vi "Host_SurfaceMetalGeneration.vi"() -> ()   [LabVIEW 2014]
uses:
  <vilib>/Instr/_visa.llb/VISA Configure Serial Port (Instr).vi
  <vilib>/FPGAPlugInAG/PCIe-7851R/niLvFpga_Open_PCIe-7851R.vi
  <vilib>/rvi/interface/common/dynamic/niFpgaDynamicAddResources.vi
  <vilib>/Utility/error.llb/Error Cluster From Error Code.vi
  <vilib>/rvi/errors/niLvFpgaAdjustHostInterfaceError.vi
  <vilib>/FPGAPlugInAG/Dynamic/niLvFpga_Close_Dynamic.vi
  <vilib>/rvi/interface/nirviOpenFPGA/nirviOpenFPGA.xnode
  FPGA Bitfiles/MetalGrowthv1_FPGATarget_FPGASurfaceSingl_DR9YibpgOIc.lvbitx
  <vilib>/rvi/interface/nirviReadWriteControl/nirviReadWriteControl.xnode
  <vilib>/rvi/interface/nirviMethod/nirviMethod.xnode
  <vilib>/rvi/interface/nirviCloseFPGA/nirviCloseFPGA.xnode
  NiFpgaLv.dll
  <vilib>/rvi/interface/Simulation/niFpgaSimulationCallBeginRW.vi
  <vilib>/FPGAPlugInAG/Dynamic/niLvFpga_ReadFifo_Dynamic.vi
  <vilib>/rvi/errors/niLvFpgaMergeErrorWithErrorCode.vi
panel:
  in  "stop":bool
  in  "DataRequired?":bool
  out "YPos":dbl
  out "XPos":dbl
  in  "XYPIZ":refnum<visa-resource-name>
  in  "GradualWithdraw?":bool
  in  "ZOffset":i32
  in  "StiffLatency":i32
  in  "ThresMultiplier":i32
  in  "OutputVoltIndex":i32
  in  "ZWithdrawStepNum":i32
  in  "ZWithdrawStepIndex":i32
  in  "ZDecStepIndex":i32
  in  "WithdrawLatency us":i32
  in  "MonitorLatency us":i32
  in  "DescendCycle":i32
  in  "YStepNum":i32
  in  "YStepLen um":dbl
  in  "YInitPos um":dbl
  in  "XInitPos um":dbl
  in  "XStepLen um":dbl
  in  "XStepNum":i32
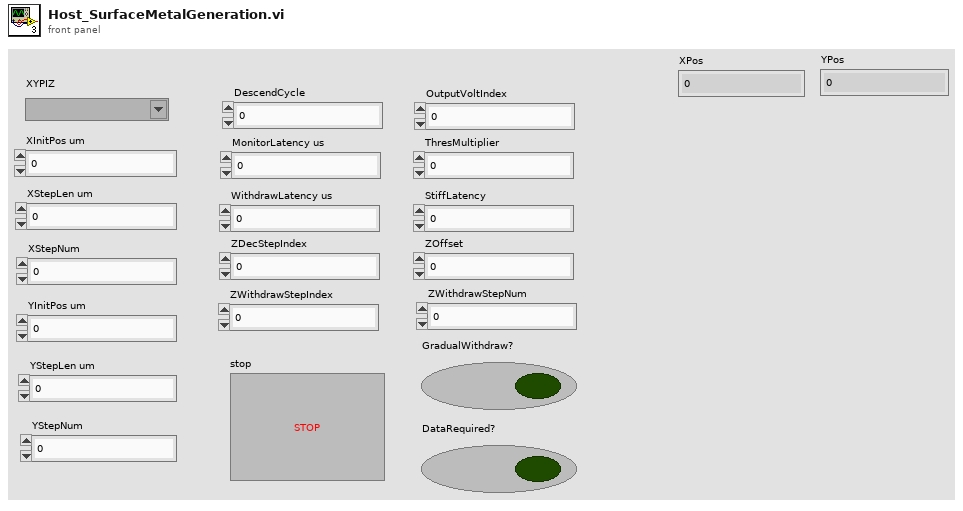
[diagram p1: front panel]
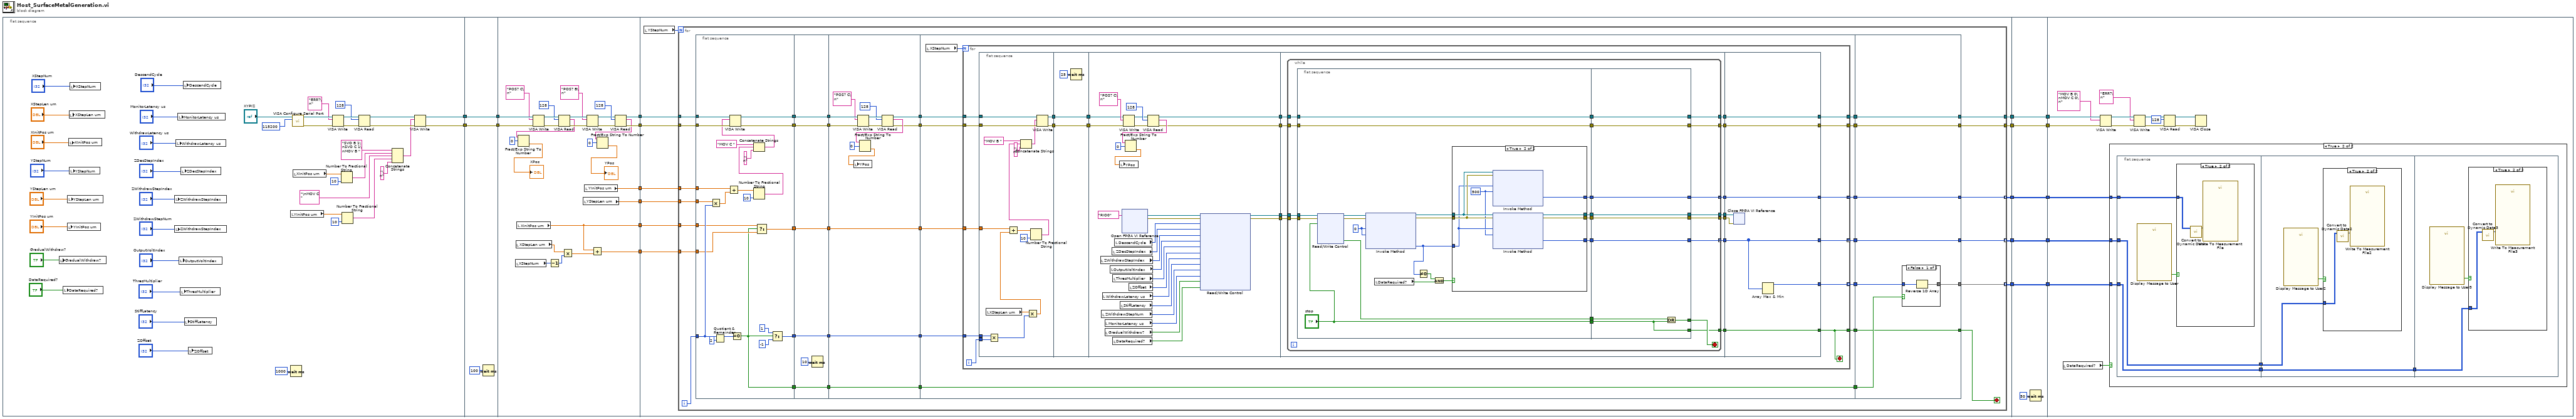
[diagram p0: block diagram]
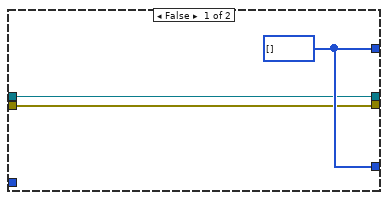
[diagram p2: hidden frame]
diagram:
  n1 = flat-sequence {
    tunnel: [w23] -> w20
    tunnel: [w22] -> w18
    tunnel: w20 -> [w63]
    tunnel: [w63] -> w19
    tunnel: w18 -> [w62]
    tunnel: [w62] -> w17
    tunnel: w19 -> [w92]
    tunnel: w17 -> [w91]
    tunnel: [w80] -> w16
    tunnel: [w79] -> w15
    tunnel: [w65] -> w14
    tunnel: [w69] -> w13
    tunnel: [w68] -> w12
    tunnel: [w67] -> w11
    tunnel: w16 -> [w100]
    tunnel: w15 -> [w99]
    tunnel: w14 -> [w103]
    tunnel: w13 -> [w102]
    tunnel: w12 -> [w101]
    tunnel: w11 -> [w98]
    tunnel: [w97] -> w10
    tunnel: [w96] -> w8
    tunnel: [w95] -> w6
    tunnel: [w94] -> w4
    tunnel: [w93] -> w2
    tunnel: w10 -> [w362]
    tunnel: [w362] -> w9
    tunnel: w8 -> [w361]
    tunnel: [w361] -> w7
    tunnel: w6 -> [w360]
    tunnel: [w360] -> w5
    tunnel: w4 -> [w359]
    tunnel: [w359] -> w3
    tunnel: w2 -> [w358]
    tunnel: [w358] -> w1
    tunnel: w9 -> [w365]
    tunnel: w7 -> [w364]
    tunnel: w5 -> [w363]
    tunnel: w3 -> [w377]
    tunnel: w1 -> [w376]
    frame #0 {
      n2 = local write "GradualWithdraw?"("GradualWithdraw?") -> ()
      n3 = local write "DataRequired?"("DataRequired?") -> ()
      n4 = local write "YInitPos um"("YInitPos um") -> ()
      n5 = local write "YStepLen um"("YStepLen um") -> ()
      n6 = local write "XInitPos um"("XInitPos um") -> ()
      n7 = local write "XStepLen um"("XStepLen um") -> ()
      n8 = local write "YStepNum"("YStepNum") -> ()
      n9 = local write "XStepNum"("XStepNum") -> ()
      n10 = local write "ZWithdrawStepIndex"("ZWithdrawStepIndex") -> ()
      n11 = local write "ZWithdrawStepIndex"("ZWithdrawStepNum") -> ()
      n12 = local write "WithdrawLatency us"("WithdrawLatency us") -> ()
      n13 = local write "MonitorLatency us"("MonitorLatency us") -> ()
      n14 = local write "OutputVoltIndex"("OutputVoltIndex") -> ()
      n15 = local write "ThresMultiplier"("ThresMultiplier") -> ()
      n16 = local write "ZDecStepIndex"("ZDecStepIndex") -> ()
      n17 = local write "DescendCycle"("DescendCycle") -> ()
      n18 = local write "StiffLatency"("StiffLatency") -> ()
      n19 = local write "ZOffset"("ZOffset") -> ()
      n20 = local read "YInitPos um"() -> (w28:dbl)
      n21 = Wait (ms)(milliseconds to wait=u32 1000) -> ()  [unwired: 1 out]
      n22 = call-poly "VISA Configure Serial Port"("VISA resource name"="XYPIZ", "baud rate (9600)"=u32 115200) -> ("VISA resource name out"=w42:refnum<visa-resource-name>, "error out"=w41:errorcluster)  [unwired: 12 in]
      n23 = local read "XInitPos um"() -> (w33:dbl)
      n24 = VISA Write(VISA resource name=w42, write buffer="ERR?\n", error in (no error)=w41) -> (VISA resource name out=w39:refnum<visa-resource-name>, error out=w38:errorcluster)  [unwired: 1 out]
      n25 = Number To Fractional String(number=w33, precision (6)=i16 10) -> (F-format string=w31:string)  [unwired: 2 in]
      n26 = Number To Fractional String(number=w28, precision (6)=i16 10) -> (F-format string=w27:string)  [unwired: 2 in]
      n27 = VISA Read(VISA resource name=w39, byte count=u32 128, error in (no error)=w38) -> (VISA resource name out=w36:refnum<visa-resource-name>, error out=w35:errorcluster)  [unwired: 2 out]
      n28 = Concatenate Strings("SVO B 1\nSVO C 1\nMOV B " ("write buffer"), w31, "\nMOV C " ("string"), w27, "\n" ("string")) -> (w25:string)
      n29 = VISA Write(VISA resource name=w36, write buffer=w25, error in (no error)=w35) -> (VISA resource name out=w23:refnum<visa-resource-name>, error out=w22:errorcluster)  [unwired: 1 out]
    }
    frame #1 {
      n30 = Wait (ms)(milliseconds to wait=u32 100) -> ()  [unwired: 1 out]
    }
    frame #2 {
      n31 = local read "XStepNum"() -> (w71:i32)
      n32 = local read "XStepLen um"() -> (w72:dbl)
      n33 = local read "XInitPos um"() -> (w65:dbl)
      n34 = VISA Write(VISA resource name=w92, write buffer="POS? C\n", error in (no error)=w91) -> (VISA resource name out=w89:refnum<visa-resource-name>, error out=w88:errorcluster)  [unwired: 1 out]
      n35 = Decrement(x=w71) -> (x-1=w70:i32)
      n36 = VISA Read(VISA resource name=w89, byte count=u32 128, error in (no error)=w88) -> (VISA resource name out=w86:refnum<visa-resource-name>, read buffer=w78:string, error out=w85:errorcluster)  [unwired: 1 out]
      n37 = Fract/Exp String To Number(string=w78, offset=0) -> (number=→"XPos":dbl)  [unwired: 2 in, 1 out]
      n38 = Multiply(x=w72, y=w70) -> (x*y=w66:dbl)
      n39 = local read "YStepLen um"() -> (w68:dbl)
      n40 = local read "YInitPos um"() -> (w67:dbl)
      n41 = VISA Write(VISA resource name=w86, write buffer="POS? B\n", error in (no error)=w85) -> (VISA resource name out=w82:refnum<visa-resource-name>, error out=w81:errorcluster)  [unwired: 1 out]
      n42 = Add(x=w65, y=w66) -> (x+y=w69:dbl)
      n43 = VISA Read(VISA resource name=w82, byte count=u32 128, error in (no error)=w81) -> (VISA resource name out=w80:refnum<visa-resource-name>, read buffer=w76:string, error out=w79:errorcluster)  [unwired: 1 out]
      n44 = Fract/Exp String To Number(string=w76, offset=0) -> (number=→"YPos":dbl)  [unwired: 2 in, 1 out]
    }
    frame #3 {
      n45 = local read "YStepNum"() -> (w104:i32)
      n46 = for {
        N: w104 -> [_]
        tunnel: w103 -> [w138]
        tunnel: w102 -> [w137]
        tunnel: w101 -> [w136]
        tunnel: w100 -> [w135]
        tunnel: w99 -> [w134]
        tunnel: w98 -> [w133]
        tunnel: [w113] -> w97 mode=indexing
        tunnel: [w112] -> w96 mode=indexing
        tunnel: [w111] -> w95 mode=indexing
        tunnel: [w108] -> w94
        tunnel: [w107] -> w93
        i -> [w139]
        stop <- w105 stop-if-true
        n47 = flat-sequence {
          tunnel: w139 -> [w157]
          tunnel: w138 -> [w151]
          tunnel: w137 -> [w150]
          tunnel: w136 -> [w158]
          tunnel: w135 -> [w160]
          tunnel: w134 -> [w159]
          tunnel: w133 -> [w155]
          tunnel: [w152] -> w132
          tunnel: [w149] -> w131
          tunnel: [w142] -> w130
          tunnel: [w141] -> w129
          tunnel: [w140] -> w119
          tunnel: w132 -> [w164]
          tunnel: w131 -> [w165]
          tunnel: w130 -> [w167]
          tunnel: w129 -> [w166]
          tunnel: [w167] -> w128
          tunnel: [w166] -> w127
          tunnel: [w165] -> w123
          tunnel: [w164] -> w121
          tunnel: [w163] -> w120
          tunnel: w119 -> [w163]
          tunnel: w128 -> [w182]
          tunnel: w127 -> [w181]
          tunnel: [w173] -> w126
          tunnel: [w172] -> w125
          tunnel: [w171] -> w124
          tunnel: w123 -> [w171]
          tunnel: [w170] -> w122
          tunnel: w121 -> [w170]
          tunnel: w120 -> [w169]
          tunnel: [w169] -> w118
          tunnel: w126 -> [w191]
          tunnel: w125 -> [w190]
          tunnel: w124 -> [w192]
          tunnel: w122 -> [w193]
          tunnel: w118 -> [w189]
          tunnel: [w189] -> w117
          tunnel: [w188] -> w116
          tunnel: [w187] -> w115
          tunnel: [w186] -> w114
          tunnel: [w185] -> w110
          tunnel: [w184] -> w109
          tunnel: [w183] -> w106
          tunnel: w117 -> [w353]
          tunnel: w116 -> [w352]
          tunnel: w115 -> [w350]
          tunnel: w114 -> [w349]
          tunnel: [w351] -> w111
          tunnel: [w350] -> w113
          tunnel: [w349] -> w112
          tunnel: w110 -> [w348]
          tunnel: w109 -> [w347]
          tunnel: [w348] -> w108
          tunnel: [w347] -> w107
          tunnel: [w346] -> w105
          tunnel: w106 -> [w346]
          frame #0 {
            n48 = Multiply(x=w158, y=w157) -> (x*y=w156:dbl)
            n49 = Quotient & Remainder(x=w157, y=2) -> (x-y*floor(x/y)=w161:i32)  [unwired: 1 out]
            n50 = Add(x=w155, y=w156) -> (x+y=w147:dbl)
            n51 = Equal To 0?(x=w161) -> (x = 0?=w140:bool)
            n52 = Number To Fractional String(number=w147, precision (6)=i16 10) -> (F-format string=w145:string)  [unwired: 2 in]
            n53 = Concatenate Strings("MOV C " ("string"), w145, "\n" ("string")) -> (w143:string)
            n54 = VISA Write(VISA resource name=w160, write buffer=w143, error in (no error)=w159) -> (VISA resource name out=w142:refnum<visa-resource-name>, error out=w141:errorcluster)  [unwired: 1 out]
            n55 = Select(t=w151, s=w140, f=w150) -> (s? t:f=w149:dbl)
            n56 = Select(t=1, s=w140, f=-1) -> (s? t:f=w152:i32)
          }
          frame #1 {
            n57 = Wait (ms)(milliseconds to wait=u32 10) -> ()  [unwired: 1 out]
          }
          frame #2 {
            n58 = VISA Write(VISA resource name=w182, write buffer="POS? C\n", error in (no error)=w181) -> (VISA resource name out=w179:refnum<visa-resource-name>, error out=w178:errorcluster)  [unwired: 1 out]
            n59 = VISA Read(VISA resource name=w179, byte count=u32 128, error in (no error)=w178) -> (VISA resource name out=w173:refnum<visa-resource-name>, read buffer=w175:string, error out=w172:errorcluster)  [unwired: 1 out]
            n60 = Fract/Exp String To Number(string=w175, offset=0) -> (number=w174:dbl)  [unwired: 2 in, 1 out]
            n61 = local write "YPos"(w174) -> ()
          }
          frame #3 {
            n62 = local read "XStepNum"() -> (w194:i32)
            n63 = for {
              N: w194 -> [_]
              tunnel: w193 -> [w220]
              tunnel: w192 -> [w218]
              tunnel: w191 -> [w217]
              tunnel: w190 -> [w216]
              tunnel: [w203] -> w188 mode=indexing
              tunnel: [w202] -> w187 mode=concatenating
              tunnel: [w201] -> w186 mode=concatenating
              tunnel: [w198] -> w185
              tunnel: [w197] -> w184
              tunnel: [w195] -> w183
              i -> [w219]
              stop <- w195 stop-if-true
              n64 = flat-sequence {
                tunnel: w220 -> [w236]
                tunnel: w219 -> [w235]
                tunnel: w218 -> [w232]
                tunnel: w217 -> [w230]
                tunnel: w216 -> [w229]
                tunnel: [w223] -> w215
                tunnel: [w222] -> w214
                tunnel: w215 -> [w238]
                tunnel: w214 -> [w237]
                tunnel: [w238] -> w213
                tunnel: [w237] -> w212
                tunnel: w213 -> [w260]
                tunnel: w212 -> [w259]
                tunnel: [w258] -> w211
                tunnel: [w257] -> w210
                tunnel: [w242] -> w209
                tunnel: [w241] -> w208
                tunnel: w211 -> [w278]
                tunnel: w210 -> [w277]
                tunnel: w209 -> [w276]
                tunnel: w208 -> [w275]
                tunnel: [w274] -> w207
                tunnel: [w273] -> w206
                tunnel: [w272] -> w205
                tunnel: [w271] -> w204
                tunnel: [w270] -> w200
                tunnel: [w269] -> w199
                tunnel: [w268] -> w196
                tunnel: w207 -> [w342]
                tunnel: w206 -> [w341]
                tunnel: w205 -> [w345]
                tunnel: w204 -> [w344]
                tunnel: [w343] -> w203
                tunnel: [w342] -> w202
                tunnel: [w341] -> w201
                tunnel: w200 -> [w340]
                tunnel: w199 -> [w339]
                tunnel: [w340] -> w198
                tunnel: [w339] -> w197
                tunnel: w196 -> [w338]
                tunnel: [w338] -> w195
                frame #0 {
                  n65 = local read "XStepLen um"() -> (w233:dbl)
                  n66 = Multiply(x=w236, y=w235) -> (x*y=w234:i32)
                  n67 = Multiply(x=w233, y=w234) -> (x*y=w231:dbl)
                  n68 = Add(x=w232, y=w231) -> (x+y=w228:dbl)
                  n69 = Number To Fractional String(number=w228, precision (6)=i16 10) -> (F-format string=w224:string)  [unwired: 2 in]
                  n70 = Concatenate Strings("MOV B " ("string"), w224, "\n" ("string")) -> (w226:string)
                  n71 = VISA Write(VISA resource name=w230, write buffer=w226, error in (no error)=w229) -> (VISA resource name out=w223:refnum<visa-resource-name>, error out=w222:errorcluster)  [unwired: 1 out]
                }
                frame #1 {
                  n72 = Wait (ms)(milliseconds to wait=u32 25) -> ()  [unwired: 1 out]
                }
                frame #2 {
                  n73 = local read "ZWithdrawStepIndex"() -> (w251:i32)
                  n74 = local read "ZWithdrawStepNum"() -> (w245:i32)
                  n75 = local read "WithdrawLatency us"() -> (w247:i32)
                  n76 = local read "MonitorLatency us"() -> (w244:i32)
                  n77 = local read "GradualWithdraw?"() -> (w243:bool)
                  n78 = local read "OutputVoltIndex"() -> (w250:i32)
                  n79 = local read "ZDecStepIndex"() -> (w252:i32)
                  n80 = local read "ThresMultiplier"() -> (w249:i32)
                  n81 = local read "DataRequired?"() -> (w240:bool)
                  n82 = local read "DescendCycle"() -> (w253:i32)
                  n83 = local read "StiffLatency"() -> (w246:i32)
                  n84 = xnode "Open FPGA VI Reference"("resource name"=tag "RIO0") -> ("FPGA VI Reference Out"=w255:refnum<k20>, "error out"=w254:errorcluster)  [unwired: 1 in]
                  n85 = VISA Write(VISA resource name=w260, write buffer="POS? C\n", error in (no error)=w259) -> (VISA resource name out=w262:refnum<visa-resource-name>, error out=w263:errorcluster)  [unwired: 1 out]
                  n86 = local read "ZOffset"() -> (w248:i32)
                  n87 = VISA Read(VISA resource name=w262, byte count=u32 128, error in (no error)=w263) -> (VISA resource name out=w258:refnum<visa-resource-name>, read buffer=w266:string, error out=w257:errorcluster)  [unwired: 1 out]
                  n88 = Fract/Exp String To Number(string=w266, offset=0) -> (number=w267:dbl)  [unwired: 2 in, 1 out]
                  n89 = local write "YPos"(w267) -> ()
                  n90 = xnode "Read/Write Control"("FPGA VI Reference In"=w255, "error in"=w254, "DescendCycle"=w253, "ZDecStepIndex"=w252, "ZWithdrawStepIndex"=w251, "OutputVoltIndex"=w250, "ThresMultiplier"=w249, "ZOffset"=w248, "WithdrawLatency us"=w247, "StiffLatency us"=w246, "ZWithdrawStepNum"=w245, "MonitorLatency us"=w244, "GradualWithdraw?"=w243, "DataRequired?"=w240) -> ("FPGA VI Reference Out"=w242:refnum<k20>, "error out"=w241:errorcluster)
                }
                frame #3 {
                  n91 = while {
                    tunnel: w278 -> [w298]
                    tunnel: w277 -> [w297]
                    tunnel: w276 -> [w296]
                    tunnel: w275 -> [w295]
                    tunnel: [w293] -> w274 mode=concatenating
                    tunnel: [w291] -> w273 mode=concatenating
                    tunnel: [w288] -> w272
                    tunnel: [w287] -> w271
                    tunnel: [w284] -> w270
                    tunnel: [w283] -> w269
                    tunnel: [w279] -> w268
                    stop <- w280 stop-if-true
                    n92 = flat-sequence {
                      tunnel: w298 -> [w302]
                      tunnel: w297 -> [w301]
                      tunnel: w296 -> [w317]
                      tunnel: w295 -> [w316]
                      tunnel: [w306] -> w294
                      tunnel: [w305] -> w292
                      tunnel: [w304] -> w290
                      tunnel: [w303] -> w289
                      tunnel: [w302] -> w286
                      tunnel: [w301] -> w285
                      tunnel: [w300] -> w282
                      tunnel: ["stop"] -> w281
                      tunnel: [w337] -> w293
                      tunnel: w294 -> [w337]
                      tunnel: w292 -> [w336]
                      tunnel: [w336] -> w291
                      tunnel: w290 -> [w335]
                      tunnel: w289 -> [w334]
                      tunnel: [w335] -> w288
                      tunnel: [w334] -> w287
                      tunnel: [w333] -> w284
                      tunnel: w286 -> [w333]
                      tunnel: [w332] -> w283
                      tunnel: w285 -> [w332]
                      tunnel: w282 -> [w331]
                      tunnel: w281 -> [w329]
                      tunnel: [w330] -> w280
                      tunnel: [w329] -> w279
                      frame #0 {
                        w313 = u32 0 ("Number of Elements")
                        n93 = xnode "Read/Write Control"("FPGA VI Reference In"=w317, "error in"=w316, "stop"="stop") -> ("FPGA VI Reference Out"=w315:refnum<k20>, "error out"=w314:errorcluster, "Finished?"=w300:bool)  [unwired: 2 out]
                        n94 = xnode "Invoke Method"("FPGA VI Reference In"=w315, "error in"=w314, "Number of Elements"=w313, "Timeout (ms)"=w313) -> ("FPGA VI Reference Out"=w312:refnum<k20>, "error out"=w311:errorcluster, "Elements Remaining"=w307:u32)  [unwired: 1 out]
                        n95 = local read "DataRequired?"() -> (w310:bool)
                        n96 = Not Equal To 0?(x=w307) -> (x != 0?=w308:bool)
                        n97 = And(x=w308, y=w310) -> (x .and. y?=w309:bool)
                        n98 = case shown="True" w309 {
                          tunnel: w312 -> [w319 w328]
                          tunnel: w311 -> [w318 w327]
                          tunnel: w307 -> [_ w326]
                          tunnel: [w320 w324] -> w306
                          tunnel: [w320 w323] -> w305
                          tunnel: [w319 w322] -> w304
                          tunnel: [w318 w321] -> w303
                          frame False {
                            w320 = i16[] [] ("Data")
                          }
                          frame True {
                            w325 = 500 ("Timeout (ms)")
                            n99 = xnode "Invoke Method"("FPGA VI Reference In"=w328, "error in"=w327, "Number of Elements"=w326, "Timeout (ms)"=w325) -> ("Data"=w324:i16[])  [unwired: 3 out]
                            n100 = xnode "Invoke Method"("FPGA VI Reference In"=w328, "error in"=w327, "Number of Elements"=w326, "Timeout (ms)"=w325) -> ("FPGA VI Reference Out"=w322:refnum<k20>, "error out"=w321:errorcluster, "Data"=w323:i16[])  [unwired: 1 out]
                          }
                        }
                      }
                      frame #1 {
                        n101 = Or(x=w331, y=w329) -> (x .or. y?=w330:bool)
                      }
                    }
                  }
                }
                frame #4 {
                  n102 = xnode "Close FPGA VI Reference"("FPGA VI Reference In"=w345, "error in"=w344) -> ()  [unwired: 1 out]
                  n103 = Array Max & Min(array=w341) -> (max value=w343:i16)  [unwired: 3 out]
                }
              }
            }
          }
          frame #4 {
            n104 = case shown="False" w353 {
              tunnel: w352 -> [w355 w356]
              tunnel: [w354 w356] -> w351
              frame False {
                n105 = Reverse 1D Array(array=w355) -> (reversed array=w354:i16[])
              }
              frame True {
              }
            }
          }
        }
      }
    }
    frame #4 {
      n106 = Wait (ms)(milliseconds to wait=u32 50) -> ()  [unwired: 1 out]
    }
    frame #5 {
      n107 = local read "DataRequired?"() -> (w366:bool)
      n108 = VISA Write(VISA resource name=w377, write buffer="MOV B 0\nMOV C 0\n", error in (no error)=w376) -> (VISA resource name out=w374:refnum<visa-resource-name>, error out=w373:errorcluster)  [unwired: 1 out]
      n109 = case shown="True" w366 {
        tunnel: w365 -> [_ w383]
        tunnel: w364 -> [_ w382]
        tunnel: w363 -> [_ w381]
        frame False {
        }
        frame True {
          n110 = flat-sequence {
            tunnel: w383 -> [w384]
            tunnel: w382 -> [w386]
            tunnel: w381 -> [w387]
            tunnel: [w387] -> w380
            tunnel: [w386] -> w379
            tunnel: w380 -> [w390]
            tunnel: w379 -> [w391]
            tunnel: [w390] -> w378
            tunnel: w378 -> [w395]
            frame #0 {
              n111 = call "Display Message to User"() -> ("OK"=w385:bool)  [unwired: 10 in, 1 out]
              n112 = case shown="True" w385 {
                tunnel: w384 -> [_ w389]
                frame False {
                }
                frame True {
                  n113 = call "Convert to Dynamic Data"("2D Array"=w389) -> ("Dynamic Data Type"=w388:dynamicdata)  [unwired: 3 in]
                  n114 = call "Write To Measurement File"("Signals"=w388) -> ()  [unwired: 16 in, 3 out]
                }
              }
            }
            frame #1 {
              n115 = call "Display Message to User2"() -> ("OK"=w392:bool)  [unwired: 10 in, 1 out]
              n116 = case shown="True" w392 {
                tunnel: w391 -> [_ w393]
                frame False {
                }
                frame True {
                  n117 = call "Convert to Dynamic Data2"("2D Array"=w393) -> ("Dynamic Data Type"=w394:dynamicdata)  [unwired: 3 in]
                  n118 = call "Write To Measurement File2"("Signals"=w394) -> ()  [unwired: 16 in, 3 out]
                }
              }
            }
            frame #2 {
              n119 = call "Display Message to User3"() -> ("OK"=w396:bool)  [unwired: 10 in, 1 out]
              n120 = case shown="True" w396 {
                tunnel: w395 -> [_ w397]
                frame False {
                }
                frame True {
                  n121 = call "Convert to Dynamic Data3"("2D Array"=w397) -> ("Dynamic Data Type"=w398:dynamicdata)  [unwired: 3 in]
                  n122 = call "Write To Measurement File3"("Signals"=w398) -> ()  [unwired: 16 in, 3 out]
                }
              }
            }
          }
        }
      }
      n123 = VISA Write(VISA resource name=w374, write buffer="ERR?\n", error in (no error)=w373) -> (VISA resource name out=w371:refnum<visa-resource-name>, error out=w370:errorcluster)  [unwired: 1 out]
      n124 = VISA Read(VISA resource name=w371, byte count=u32 128, error in (no error)=w370) -> (VISA resource name out=w368:refnum<visa-resource-name>, error out=w367:errorcluster)  [unwired: 2 out]
      n125 = VISA Close(VISA resource name=w368, error in (no error)=w367) -> ()  [unwired: 1 out]
    }
  }
